vi "Break_down_indicator_status.vi"(10 "Array":bool[](array[boolean]), 11 "Cluster in":refnum<vi>) -> (3 "Controls[]":refnum<vi>[](array[refnum]))   [LabVIEW 2017]
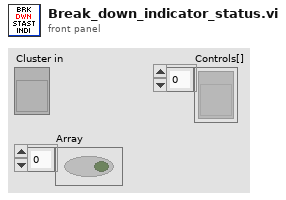
[diagram p1: front panel]
types:
  T1 = cluster{"Array[0]":bool, "Array[1]":bool, "Array[2]":bool, "Array[3]":bool, "Array[4]":bool}
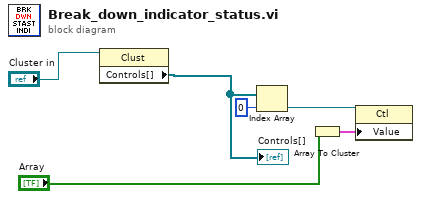
[diagram p0: block diagram]
diagram:
  n1 = property on="Property Node" class="Clust"(reference="Cluster in") -> ("Controls[]"=w6:refnum<vi>[])  [unwired: 1 in, 2 out]
  "Controls[]" <- w6
  n2 = Index Array(array=w6, index=0) -> (element=w4:refnum<vi>)
  n3 = Array To Cluster(array="Array") -> (cluster=w1:T1)
  n4 = property class="Ctl"(reference=w4, "Value"=w1) -> ()  [unwired: 1 in, 2 out]
